vi "Add Items.vi"(7 "Mode":enum16{"End", "Begin"}(ring), 8 "错误输入":errorcluster, 10 "Items":string[](array[string]), 11 "Listbox Ref":refnum<vi>) -> (0 "错误输出":errorcluster, 3 "Dup Listbox Ref":refnum<vi>)   [LabVIEW 2012, in "Listbox Tool.lvlib"]
uses:
  Listbox Tool.lvlib
  Custom Type/Read and Write Mode.ctl
  Property/Set and Get ItemNames.vi
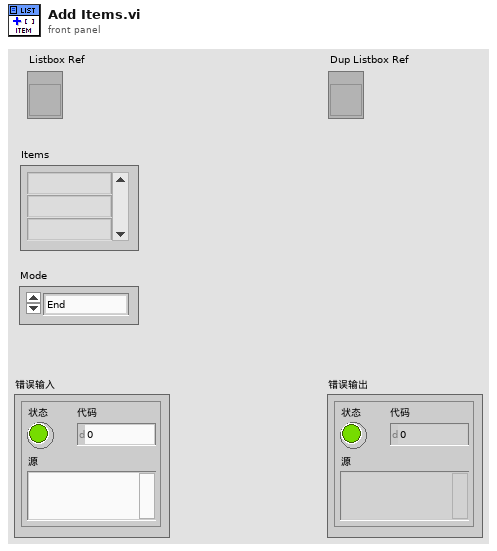
[diagram p1: front panel]
types:
  T1 = typedef "Listbox Tool.lvlib/Read and Write Mode.ctl" = enum16{"Read", "Write"}
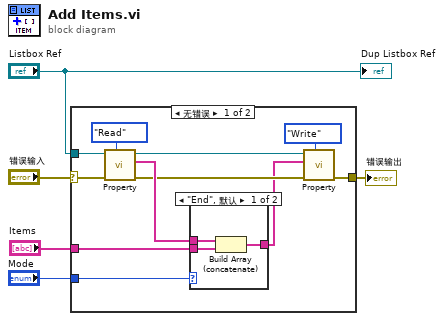
[diagram p0: block diagram]
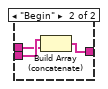
[diagram p2: hidden frame]
diagram:
  n1 = case shown="无错误" "错误输入" {
    selector: "错误输入" -> [w16 w23]
    tunnel: "Listbox Ref" -> [w15 _]
    tunnel: "Items" -> [w13 _]
    tunnel: "Mode" -> [w9 _]
    tunnel: [w8 w23] -> w1
    frame No Error {
      n2 = call-poly "Property.vi"("Mode"=Read_and_Write_Mode."Read", "错误输入"=w16, "Listbox Ref"=w15) -> ("错误输出"=w12:errorcluster, "ItemNames Out"=w14:string[], "Dup Listbox Ref"=w11:refnum<vi>)  [unwired: 6 in]
      n3 = case shown="\"End\", 默认" w9 {
        tunnel: w14 -> [w19 w21]
        tunnel: w13 -> [w18 w22]
        tunnel: [w17 w20] -> w7
        frame "End", Default {
          n4 = Build Array (concatenate)(w19, w18) -> (w17:string[])
        }
        frame "Begin" {
          n5 = Build Array (concatenate)(w22, w21) -> (w20:string[])
        }
      }
      n6 = call-poly "Property.vi"("Mode"=Read_and_Write_Mode."Write", "错误输入"=w12, "ItemNames In"=w7, "Listbox Ref"=w11) -> ("错误输出"=w8:errorcluster)  [unwired: 5 in, 2 out]
    }
    frame Error {
    }
  }
  "错误输出" <- w1
  "Dup Listbox Ref" <- "Listbox Ref"
